vi "Word Add New Document.vi"(0 "report in":refnum<class "NI_report.lvclass">, 7 "document path (not a path)":path, 11 "error in (no error)":errorcluster) -> (4 "report out":refnum<class "NI_report.lvclass">, 15 "error out":errorcluster)   [LabVIEW 2010, in "NI_Word.lvclass"]
doc: "Adds a new document to the document collection."
uses:
  <vilib>/Utility/NIReport.llb/Word/NI_Word.lvclass
  <vilib>/Utility/NIReport.llb/NI_report.lvclass
  <vilib>/Utility/NIReport.llb/Word/NI_Word.lvclass/NI_Word.ctl
  <vilib>/Utility/NIReport.llb/NI_ReportGenerationCore.lvlib
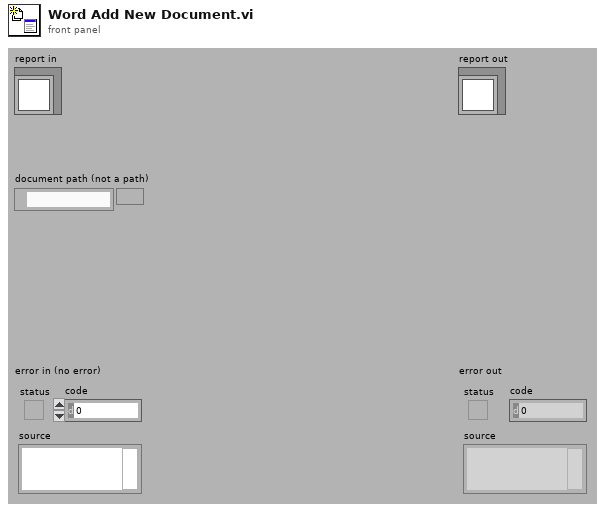
[diagram p1: front panel]
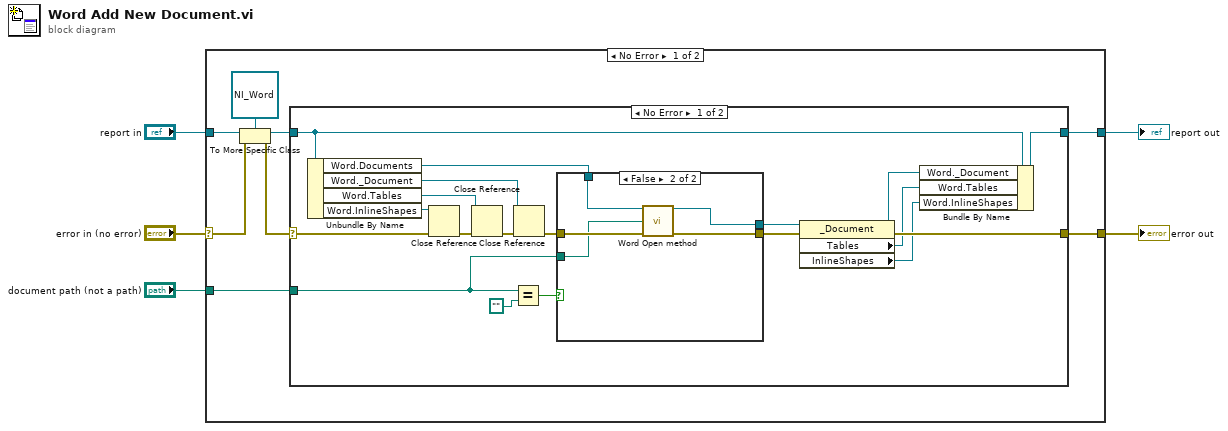
[diagram p0: block diagram]
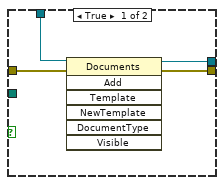
[diagram p2: hidden frame]
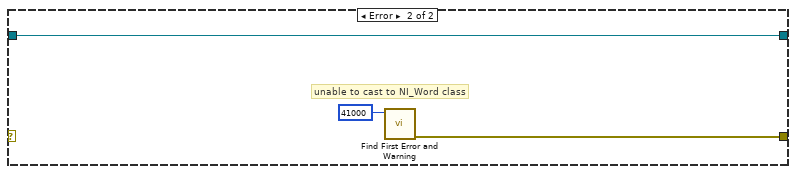
[diagram p3: hidden frame]
diagram:
  n1 = case shown="No Error" "error in (no error)" {
    selector: "error in (no error)" -> [w6 w46]
    tunnel: [w13 w46] -> w4
    tunnel: [w12 w45] -> w2
    tunnel: "report in" -> [w9 w45]
    tunnel: "document path (not a path)" -> [w11 _]
    frame No Error {
      n2 = To More Specific Class(target class=refnum<class "NI_Word.lvclass"> refnum ("report in"), reference=w9, error in=w6) -> (specific class reference=w8:refnum<class "NI_Word.lvclass">, error out=w7:errorcluster)
      n3 = case shown="No Error" w7 {
        selector: w7 -> [w17 _]
        tunnel: [w20 w42] -> w13
        tunnel: [w19 w44] -> w12
        tunnel: w11 -> [w14 _]
        tunnel: w8 -> [w18 w44]
        frame No Error {
          n4 = Unbundle By Name(w18) -> ("Word.Documents"=w21:refnum<k7>, "Word._Document"=w31:refnum<k7>, "Word.Tables"=w30:refnum<k7>, "Word.InlineShapes"=w29:refnum<k7>)
          n5 = Close Reference(reference=w29, error in (no error)=w17) -> (error out=w26:errorcluster)
          n6 = Close Reference(reference=w30, error in (no error)=w26) -> (error out=w27:errorcluster)
          n7 = Equal?(x=w14, y=path "") -> (x = y?=w25:bool)
          n8 = Close Reference(reference=w31, error in (no error)=w27) -> (error out=w28:errorcluster)
          n9 = case shown="False" w25 {
            tunnel: w21 -> [w36 w39]
            tunnel: w28 -> [w35 w38]
            tunnel: [w34 w41] -> w22
            tunnel: [w33 w40] -> w32
            tunnel: w14 -> [_ w37]
            frame True {
              n10 = invoke class="Documents" method="Add"(reference=w36, error in=w35) -> (error out=w33:errorcluster, "Add"=w34:refnum<k7>)  [unwired: 5 in, 5 out]
            }
            frame False {
              n11 = call <vilib>:"Word Open method.vi"("Word.Documents"=w39, "FileName"=w37, "error in (no error)"=w38) -> ("Open"=w41:refnum<k7>, "error out"=w40:errorcluster)  [unwired: 11 out]
            }
          }
          n12 = property class="_Document"(reference=w22, error in=w32) -> (reference out=w23:refnum<k7>, error out=w20:errorcluster, "Tables"=w16:refnum<k7>, "InlineShapes"=w15:refnum<k7>)
          n13 = Bundle By Name(cluster=w18, "Word._Document"=w23, "Word.Tables"=w16, "Word.InlineShapes"=w15) -> (w19:refnum<class "NI_Word.lvclass">)
        }
        frame Error {
          # "unable to cast to NI_Word class"
          n14 = call <vilib>:"Find First Error and Warning.vi"("error code"=41000) -> ("error out"=w42:errorcluster)  [unwired: 2 in, 4 out]
        }
      }
    }
    frame Error {
    }
  }
  "error out" <- w4
  "report out" <- w2
